vi "RPC__method Template.vi"(8 "error in (no error)":errorcluster, 11 "OOP Server in":refnum<class "Template Server.lvclass">) -> (0 "error out":errorcluster, 3 "OOP Server out":refnum<class "Template Server.lvclass">)   [LabVIEW 2019, in "Template Server.lvlib" / "Template Server.lvclass"]
uses:
  Template Server.lvclass
  Template Server.lvclass/Template Server.ctl
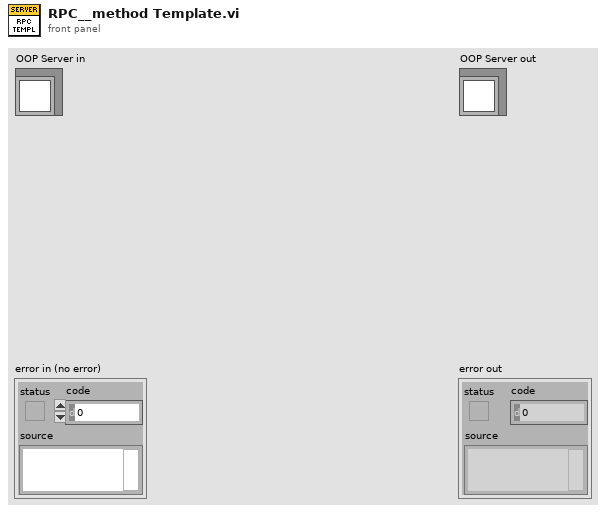
[diagram p1: front panel]
types:
  T1 = typedef "Template Server.lvlib/Template Server.lvclass/Server Internal UEs.ctl" = cluster{"Template Internal UE":T2}
  T2 = typedef "Template Server.lvlib/Template Server.lvclass/Server Internal Data UE.ctl" = refnum<user-event>
  T3 = typedef "Template Server.lvlib/Template Server.lvclass/Server gRPC UEs.ctl" = cluster{"Template gRPCId UE":T4}
  T4 = typedef "Template Server.lvlib/gprc-lvsupport.lvlib/gRPCId Cluster UE.ctl" = refnum<user-event>
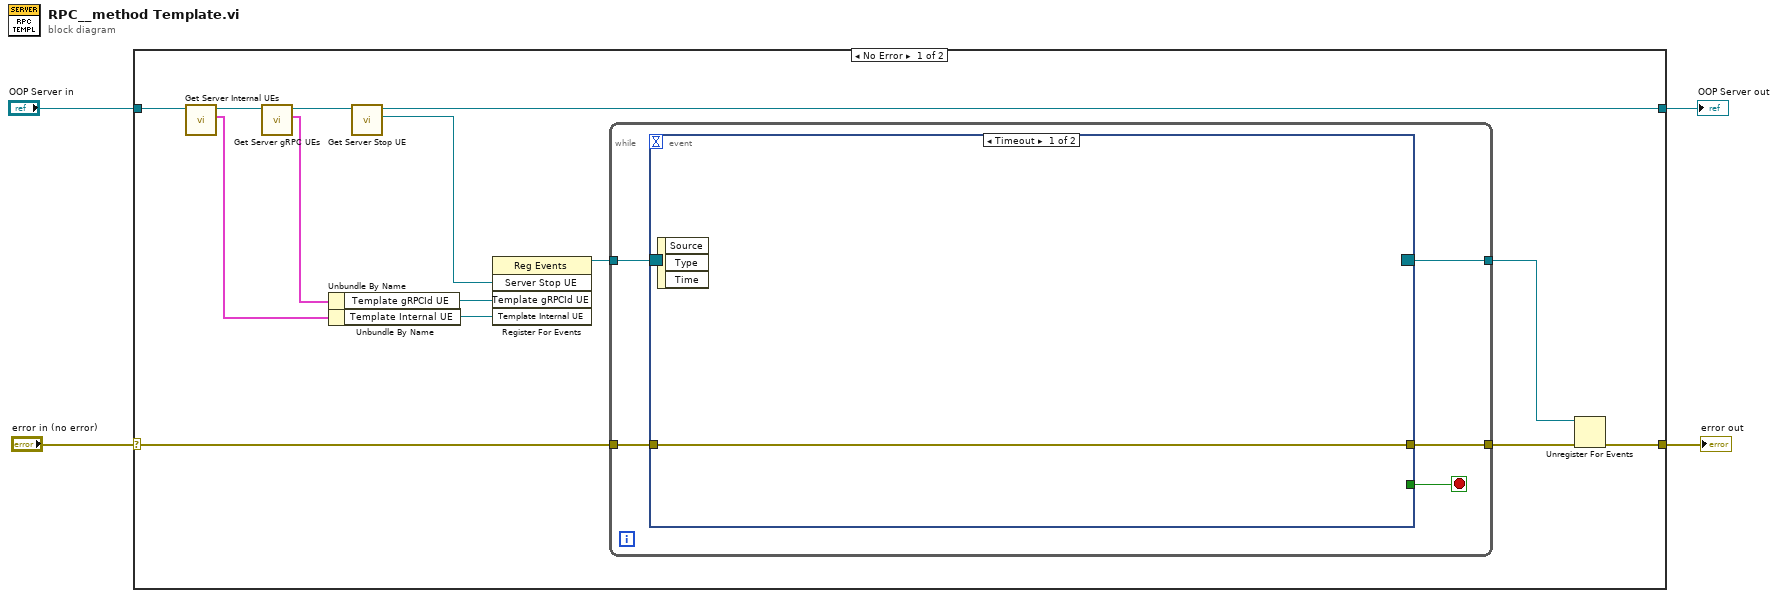
[diagram p0: block diagram]
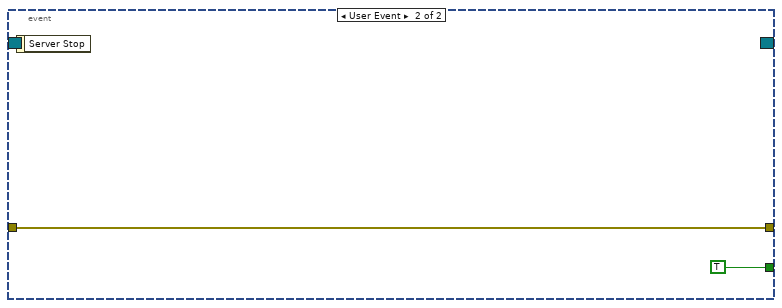
[diagram p2: hidden frame]
diagram:
  n1 = case shown="No Error" "error in (no error)" {
    selector: "error in (no error)" -> [w12 w28]
    tunnel: [w10 w28] -> w3
    tunnel: [w16 w27] -> w1
    tunnel: "OOP Server in" -> [w14 w27]
    frame No Error {
      n2 = call "Get Server Internal UEs.vi"("OOP Server in"=w14) -> ("Server Internal UEs"=w6:T1, "OOP Server out"=w13:refnum<class "Template Server.lvclass">)  [unwired: 9 in]
      n3 = call "Get Server gRPC UEs.vi"("OOP Server in"=w13) -> ("Server gRPC UEs"=w8:T3, "OOP Server out"=w18:refnum<class "Template Server.lvclass">)  [unwired: 9 in]
      n4 = Unbundle By Name(w8) -> ("Template gRPCId UE"=w7:T4)
      n5 = Unbundle By Name(w6) -> ("Template Internal UE"=w5:T2)
      n6 = call "Get Server Stop UE.vi"("OOP Server in"=w18) -> ("Server Stop UE"=w17:refnum<user-event>, "OOP Server out"=w16:refnum<class "Template Server.lvclass">)  [unwired: 9 in]
      n7 = register-events(w17, w7, w5) -> (reference out=w15:refnum<event-registration>)  [unwired: 2 in, 1 out]
      n8 = while {
        tunnel: w15 -> [w23]
        tunnel: w12 -> [w21]
        tunnel: [w20] -> w11
        tunnel: [w19] -> w9
        stop <- w22 stop-if-true
        n9 = event shown="[0] Timeout" {
          selector: w23 -> [_ _]
          dyn-events: [_ _] -> w19
          timeout: _ -> [_ _]
          tunnel: [_ TRUE] -> w22
          tunnel: w21 -> [w24 w25]
          tunnel: [w24 w25] -> w20
          event Timeout {
            n10 = event-data() -> ()  [unwired: 1 in, 3 out]
          }
          event User Event {
            n11 = event-data() -> ()  [unwired: 1 in, 1 out]
          }
        }
      }
      n12 = Unregister For Events(event registration refnum=w9, error in=w11) -> (error out=w10:errorcluster)
    }
    frame Error {
    }
  }
  "error out" <- w3
  "OOP Server out" <- w1
